vi "RunBotSpeak.vi"(3 "VIA":path=path "/Kim/Users/crogers/Documents/LabVIEW Data/LVVIAGenerated/Demo1.vi  2013-12-18 14-09-36.via") -> (1 "BotSpeak":string)   [LabVIEW 2014]
panel:
  out "text":string
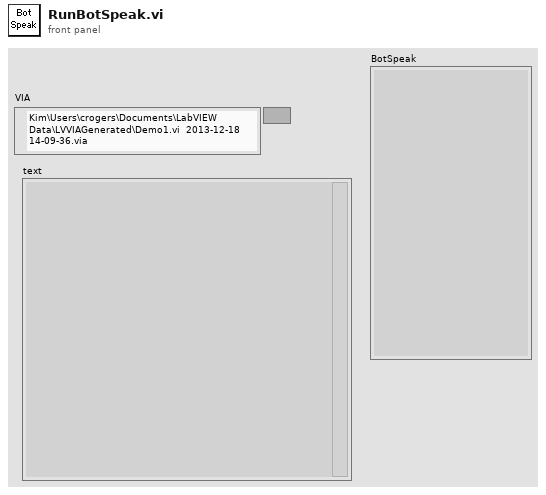
[diagram p1: front panel]
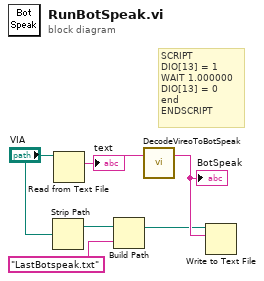
[diagram p0: block diagram]
diagram:
  # "SCRIPT\nDIO[13] = 1\nWAIT 1.000000\nDIO[13] = 0\nend\nENDSCRIPT"
  n1 = Strip Path(path="VIA") -> (stripped path=w4:path)  [unwired: 1 out]
  n2 = Read from Text File(file (use dialog)="VIA") -> (text=w6:string)  [unwired: 3 in, 3 out]
  "text" <- w6
  n3 = Build Path(base path=w4, name or relative path="LastBotspeak.txt") -> (appended path=w1:path)
  n4 = call <vilib>:"DecodeVireoToBotSpeak.vi"("Via file"=w6) -> ("BotSpeak"=w2:string)  [unwired: 2 in]
  "BotSpeak" <- w2
  n5 = Write to Text File(file (use dialog)=w1, text=w2) -> ()  [unwired: 2 in, 3 out]
